vi "Set ItemID.vi"(8 "error in (no error)":errorcluster, 11 "SM EOL Station Actor in":refnum<class "OPC Server.lvclass">) -> (0 "error out":errorcluster, 3 "SM EOL Station Actor out":refnum<class "OPC Server.lvclass">)   [LabVIEW 2021]
uses:
  <vilib>/OPCUA/controls/Data Type.ctl
  <vilib>/OPCUA/NI OPC UA Server.lvlib
  OPC Server.lvclass
  C:/Program Files/National Instruments/LabVIEW 2021/vi.lib/ActorFramework/Actor/Actor.lvclass
  C:/GitHub/SM EOL OPC Server AF/SM EOL Station Actor/SM EOL Station Actor/OPC Server.lvclass
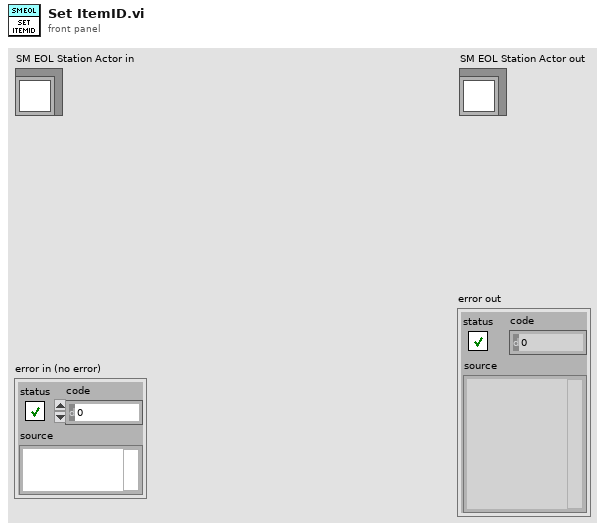
[diagram p1: front panel]
types:
  T1 = typedef "Data Type.ctl" = u16
  T2 = cluster{"name":string, "data type":T1, "access level":u16, "description":string}
  T3 = typedef "NodeId.ctl" = string
  T4 = typedef "OPC UA Server Refnum.ctl" = refnum<k21>
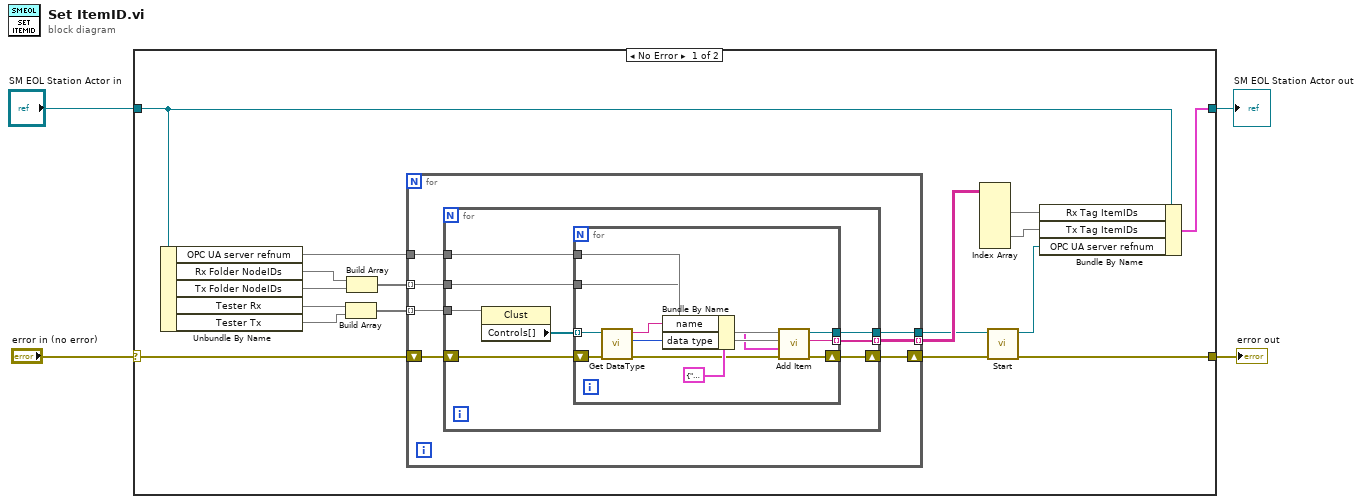
[diagram p0: block diagram]
diagram:
  n1 = case shown="No Error" "error in (no error)" {
    selector: "error in (no error)" -> [w21 w50]
    tunnel: [w7 w50] -> w3
    tunnel: [w12 w49] -> w1
    tunnel: "SM EOL Station Actor in" -> [w19 w49]
    frame No Error {
      n2 = Unbundle By Name(w19) -> ("OPC UA server refnum"=w20, "Rx Folder NodeIDs"=w15, "Tx Folder NodeIDs"=w14, "Tester Rx"=w18, "Tester Tx"=w17)
      n3 = Build Array(w18, w17) -> (w16:void[])
      n4 = Build Array(w15, w14) -> (w13:void[])
      n5 = for {
        tunnel: w16 -> [w26] mode=indexing
        tunnel: w13 -> [w25] mode=indexing
        tunnel: w20 -> [w24]
        tunnel: [w23] -> w11 mode=indexing
        shift-right: [w27] -> w8
        shift-left: w21 -> [w28]
        tunnel: [w22] -> w6
        n6 = for {
          tunnel: w25 -> [w35]
          tunnel: [w32] -> w23 mode=indexing
          tunnel: w26 -> [w31]
          shift-right: [w34] -> w27
          shift-left: w28 -> [w36]
          tunnel: w24 -> [w33]
          tunnel: [w29] -> w22
          n7 = property class="Clust"(reference=w31) -> ("Controls[]"=w30:refnum<vi>[])  [unwired: 1 in, 2 out]
          n8 = for {
            tunnel: w33 -> [w48]
            tunnel: w35 -> [w47]
            shift-right: [w46] -> w34
            shift-left: w36 -> [w41]
            tunnel: [w45] -> w32 mode=indexing
            tunnel: w30 -> [w42] mode=indexing
            tunnel: [w37] -> w29
            n9 = call "Get DataType.vi"("error in (no error)"=w41, "reference"=w42) -> ("error out"=w39:errorcluster, "data type"=w38:T1, "Name"=w40:string)  [unwired: 7 in]
            n10 = Bundle By Name(cluster=T2 {"name"="", "data type"=1, "access level"=3, "description"=""} ("item"), "name"=w40, "data type"=w38) -> (w43:T2)
            n11 = call <vilib>:"Add Item.vi"("error in (no error)"=w39, "item"=w43, "parent folder node ID"=w47, "OPC UA server refnum in"=w48) -> ("error out"=w46:errorcluster, "item node ID"=w45:T3, "OPC UA server refnum out"=w37:T4)  [unwired: 3 in, 1 out]
          }
        }
      }
      n12 = Index Array(array=w11) -> (element #1=w10:T3[][], element #2=w9:T3[][])  [unwired: 6 in]
      n13 = call <vilib>:"Start.vi"("error in (no error)"=w8, "OPC UA server refnum in"=w6) -> ("error out"=w7:errorcluster, "OPC UA server refnum out"=w5:T4)  [unwired: 7 in, 1 out]
      n14 = Bundle By Name(cluster=w19, "Rx Tag ItemIDs"=w10, "Tx Tag ItemIDs"=w9, "OPC UA server refnum"=w5) -> (w12:cluster{})
    }
    frame Error {
    }
  }
  "error out" <- w3
  "SM EOL Station Actor out" <- w1
